vi "RUSHArmControl.vi"(1 "In Cluster":T3) -> (0 "Out Cluster":T2)   [LabVIEW 2012]
uses:
  <vilib>/Rock Robotics/WPI/Relay/WPI_RelayValue.ctl
panel:
  in  "Setpoint P Gain":dbl=2.0
  in  "Manual P Gain":dbl=2.0
  in  "Vision P Gain":dbl=0.75
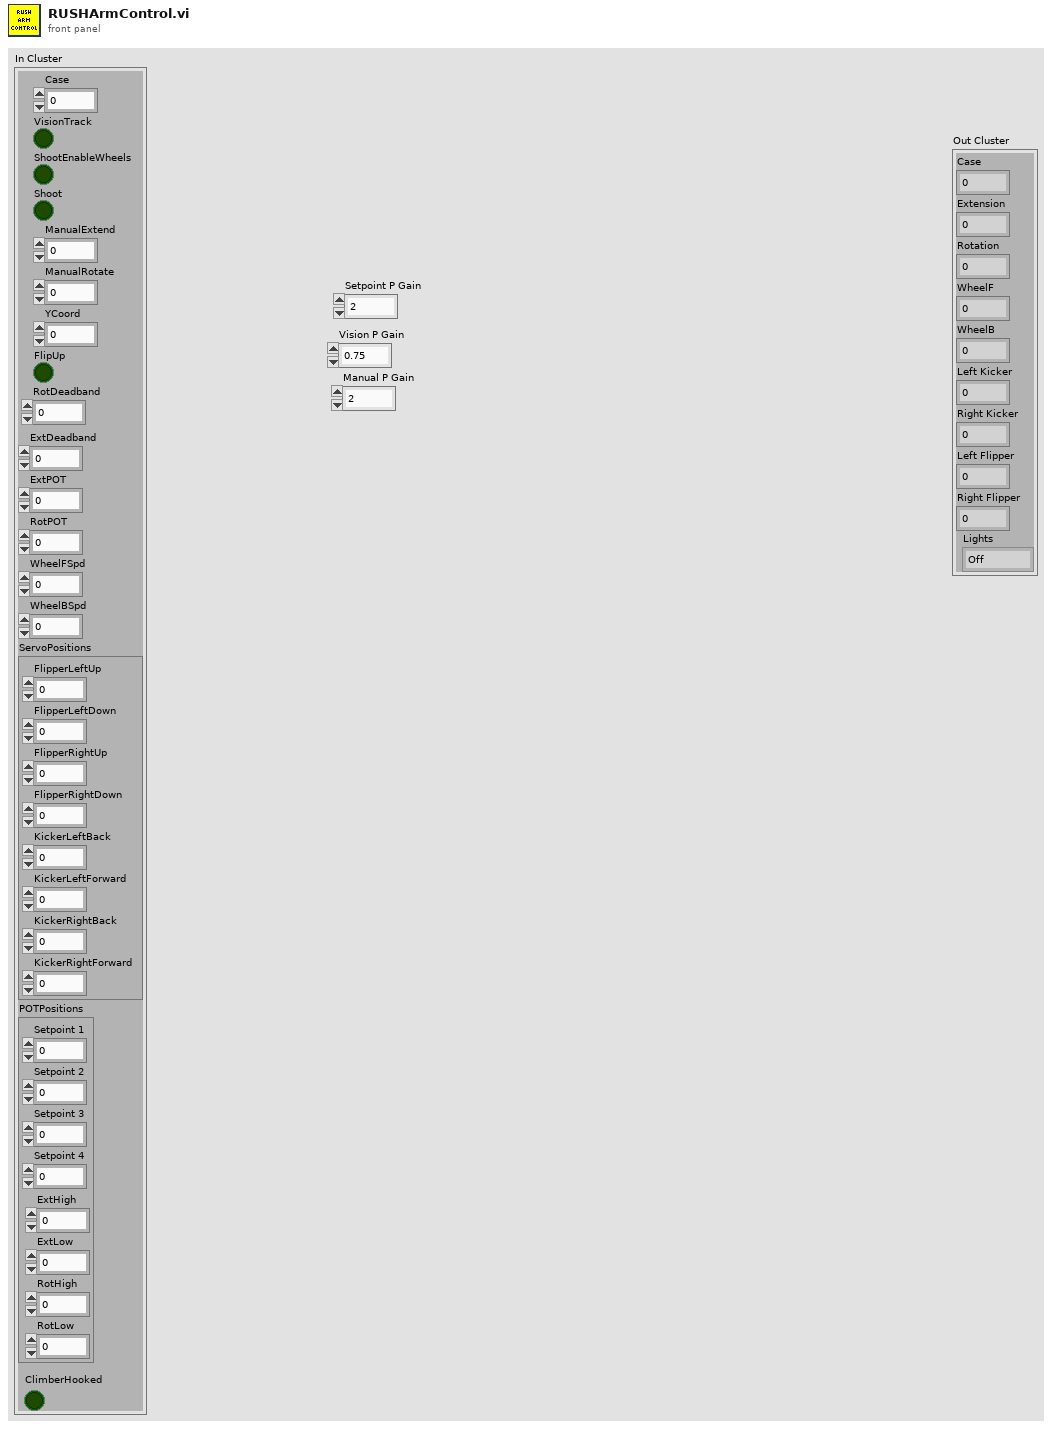
[diagram p1: front panel]
types:
  T1 = typedef "WPI_RelayValue.ctl" = enum16{"Off", "On", "Forward", "Reverse"}
  T2 = cluster{"Case":dbl, "Extension":dbl, "Rotation":dbl, "WheelF":dbl, "WheelB":dbl, "Left Kicker":dbl, "Right Kicker":dbl, "Left Flipper":dbl, "Right Flipper":dbl, "Lights":T1}
  T3 = cluster{"Case":dbl, "VisionTrack":bool, "ShootEnableWheels":bool, "Shoot":bool, "ManualExtend":dbl, "ManualRotate":dbl, "YCoord":dbl, "FlipUp":bool, "RotDeadband":dbl, "ExtDeadband":dbl, "ExtPOT":dbl, "RotPOT":dbl, "WheelFSpd":dbl, "WheelBSpd":dbl, "ServoPositions":cluster{"FlipperLeftUp":dbl, "FlipperLeftDown":dbl, "FlipperRightUp":dbl, "FlipperRightDown":dbl, "KickerLeftBack":dbl, "KickerLeftForward":dbl, "KickerRightBack":dbl, "KickerRightForward":dbl}, "POTPositions":cluster{"Setpoint 1":dbl, "Setpoint 2":dbl, "Setpoint 3":dbl, "Setpoint 4":dbl, "RotLow":dbl, "RotHigh":dbl, "ExtLow":dbl, "ExtHigh":dbl}, "ClimberHooked":bool}
  T4 = cluster{"FlipperLeftUp":dbl, "FlipperLeftDown":dbl, "FlipperRightUp":dbl, "FlipperRightDown":dbl, "KickerLeftBack":dbl, "KickerLeftForward":dbl, "KickerRightBack":dbl, "KickerRightForward":dbl}
  T5 = cluster{"Setpoint 1":dbl, "Setpoint 2":dbl, "Setpoint 3":dbl, "Setpoint 4":dbl, "RotLow":dbl, "RotHigh":dbl, "ExtLow":dbl, "ExtHigh":dbl}
  T6 = cluster{"t":dbl, "y":dbl, "y":dbl, "Output":dbl, "Output":dbl, "KickerLeftBack":dbl, "KickerRightBack":dbl, "FlipperLeftDown":dbl, "FlipperRightDown":dbl, "RelayValue":T1}
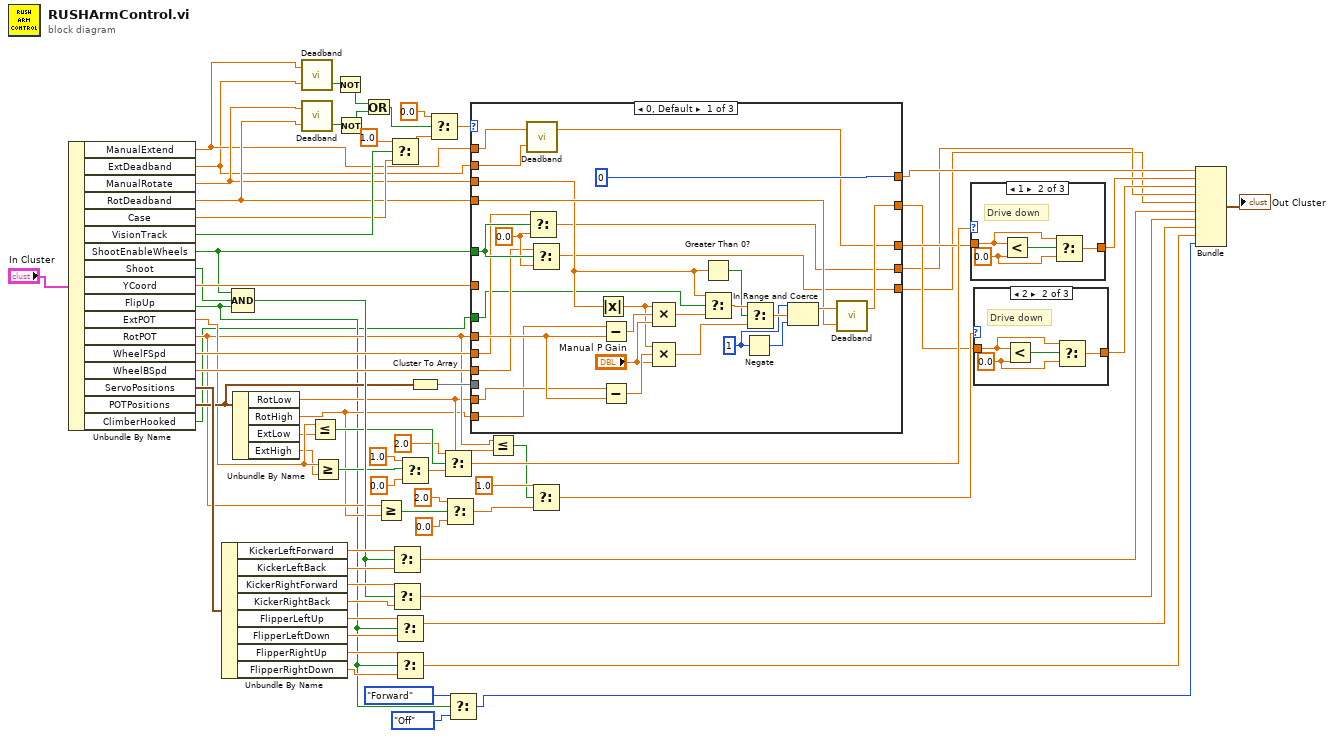
[diagram p0: block diagram]
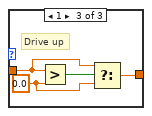
[diagram p3: hidden frame]
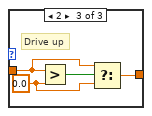
[diagram p5: hidden frame]
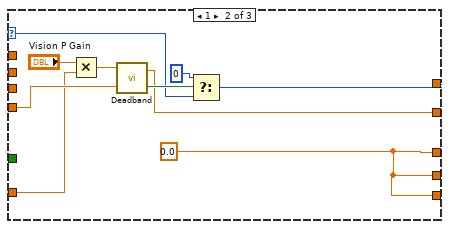
[diagram p6: hidden frame]
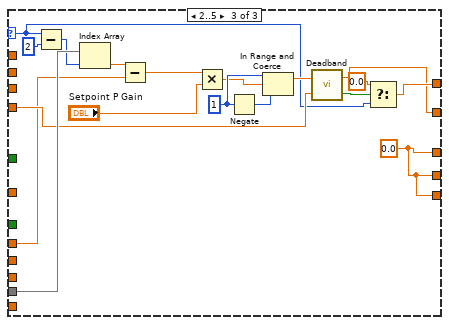
[diagram p7: hidden frame]
diagram:
  n1 = Unbundle By Name("In Cluster") -> ("ManualExtend"=w55:dbl, "ExtDeadband"=w54:dbl, "ManualRotate"=w56:dbl, "RotDeadband"=w58:dbl, "Case"=w59:dbl, "VisionTrack"=w60:bool, "ShootEnableWheels"=w49:bool, "Shoot"=w50:bool, "YCoord"=w57:dbl, "FlipUp"=w5:bool, "ExtPOT"=w32:dbl, "RotPOT"=w20:dbl, "WheelFSpd"=w53:dbl, "WheelBSpd"=w52:dbl, "ServoPositions"=w51:T4, "POTPositions"=w39:T5, "ClimberHooked"=w3:bool)
  n2 = Unbundle By Name(w51) -> ("KickerLeftForward"=w48:dbl, "KickerLeftBack"=w47:dbl, "KickerRightForward"=w46:dbl, "KickerRightBack"=w45:dbl, "FlipperLeftUp"=w43:dbl, "FlipperLeftDown"=w41:dbl, "FlipperRightUp"=w42:dbl, "FlipperRightDown"=w40:dbl)
  n3 = Compound Arithmetic op=AND(w49, w50, w5) -> (w44:bool)
  n4 = Unbundle By Name(w39) -> ("RotLow"=w19:dbl, "RotHigh"=w18:dbl, "ExtLow"=w31:dbl, "ExtHigh"=w30:dbl)
  n5 = call "Deadband.vi"("Deadband"=w54, "Input"=w55) -> ("In Deadband"=w65:bool)  [unwired: 1 out]
  n6 = call "Deadband.vi"("Deadband"=w58, "Input"=w56) -> ("In Deadband"=w64:bool)  [unwired: 1 out]
  n7 = Less Or Equal?(x=w32, y=w31) -> (x <= y?=w33:bool)
  n8 = Greater Or Equal?(x=w32, y=w30) -> (x >= y?=w37:bool)
  n9 = Not(x=w65) -> (.not. x?=w62:bool)
  n10 = Not(x=w64) -> (.not. x?=w63:bool)
  n11 = Or(x=w62, y=w63) -> (x .or. y?=w61:bool)
  n12 = Greater Or Equal?(x=w20, y=w18) -> (x >= y?=w21:bool)
  n13 = Select(t=1.0, s=w60, f=w59) -> (s? t:f=w67:dbl)
  n14 = Select(t=w48, s=w44, f=w47) -> (s? t:f=w10:dbl)
  n15 = Select(t=w46, s=w44, f=w45) -> (s? t:f=w9:dbl)
  n16 = Select(t=w43, s=w5, f=w41) -> (s? t:f=w8:dbl)
  n17 = Select(t=w42, s=w5, f=w40) -> (s? t:f=w7:dbl)
  n18 = Select(t=1.0, s=w37, f=0.0) -> (s? t:f=w34:dbl)
  n19 = Cluster To Array(cluster=w39) -> (array=w38:dbl[])
  n20 = Select(t=0.0, s=w61, f=w67) -> (s? t:f=w70:dbl)
  n21 = Select(t=2.0, s=w33, f=w34) -> (s? t:f=w28:dbl)
  n22 = Select(t=2.0, s=w21, f=0.0) -> (s? t:f=w24:dbl)
  n23 = Select(t=WPI_RelayValue."Forward" ("RelayValue"), s=w5, f=WPI_RelayValue."Off" ("RelayValue")) -> (s? t:f=w1:T1)
  n24 = case shown="0, Default" w70 {
    selector: w70 -> [_ w104 w113]
    tunnel: w58 -> [w84 w107 w117]
    tunnel: w57 -> [_ w106 _]
    tunnel: [0 ("t") w102 w112] -> w15
    tunnel: [w82 w101 w111] -> w16
    tunnel: w20 -> [w87 _ w116]
    tunnel: w19 -> [w86 _ _]
    tunnel: w18 -> [w85 _ _]
    tunnel: w56 -> [w83 _ _]
    tunnel: w55 -> [w80 _ _]
    tunnel: w54 -> [w79 _ _]
    tunnel: [w78 w100 w110] -> w27
    tunnel: w49 -> [w77 _ _]
    tunnel: w53 -> [w75 _ _]
    tunnel: w52 -> [w74 _ _]
    tunnel: [w73 w100 w110] -> w12
    tunnel: [w72 w100 w110] -> w11
    tunnel: w38 -> [_ _ w126]
    tunnel: w3 -> [w71 _ _]
    frame 0, Default {
      w76 = 0.0 ("f")
      w89 = 1
      n25 = call "Deadband.vi"("Deadband"=w79, "Input"=w80) -> ("Output"=w78:dbl)  [unwired: 1 out]
      n26 = Select(t=w75, s=w77, f=w76) -> (s? t:f=w73:dbl)
      n27 = Select(t=w74, s=w77, f=w76) -> (s? t:f=w72:dbl)
      n28 = Absolute Value(x=w83) -> (abs(x)=w93:dbl)
      n29 = Subtract(x=w85, y=w87) -> (x-y=w99:dbl)
      n30 = Subtract(x=w86, y=w87) -> (x-y=w98:dbl)
      n31 = Compound Arithmetic op=MULTIPLY(w93, w99, "Manual P Gain") -> (w96:dbl)
      n32 = Compound Arithmetic op=MULTIPLY(w93, w98, "Manual P Gain") -> (w94:dbl)
      n33 = Greater Than 0?(x=w83) -> (x > 0?=w92:bool)
      n34 = Select(t=w83, s=w71, f=w96) -> (s? t:f=w95:dbl)
      n35 = Negate(x=w89) -> (-x=w90:i32)
      n36 = Select(t=w95, s=w92, f=w94) -> (s? t:f=w91:dbl)
      n37 = In Range and Coerce(upper limit=w89, x=w91, lower limit=w90) -> (coerced(x)=w88:dbl)  [unwired: 1 out]
      n38 = call "Deadband.vi"("Deadband"=w84, "Input"=w88) -> ("Output"=w82:dbl)  [unwired: 1 out]
    }
    frame 1 {
      w100 = 0.0 ("Output")
      n39 = Multiply(x="Vision P Gain", y=w106) -> (x*y=w108:dbl)
      n40 = call "Deadband.vi"("Deadband"=w107, "Input"=w108) -> ("In Deadband"=w105:bool, "Output"=w101:dbl)
      n41 = Select(t=0, s=w105, f=w104) -> (s? t:f=w102:i32)
    }
    frame 2..5 {
      w110 = 0.0 ("Output")
      w120 = 1
      n42 = Subtract(x=w113, y=2) -> (x-y=w125:i32)
      n43 = Index Array(array=w126, index=w125) -> (element=w124:dbl)
      n44 = Subtract(x=w124, y=w116) -> (x-y=w123:dbl)
      n45 = Multiply(x=w123, y="Setpoint P Gain") -> (x*y=w119:dbl)
      n46 = Negate(x=w120) -> (-x=w121:i32)
      n47 = In Range and Coerce(upper limit=w120, x=w119, lower limit=w121) -> (coerced(x)=w118:dbl)  [unwired: 1 out]
      n48 = call "Deadband.vi"("Deadband"=w117, "Input"=w118) -> ("In Deadband"=w115:bool, "Output"=w111:dbl)
      n49 = Select(t=0.0, s=w115, f=w113) -> (s? t:f=w112:dbl)
    }
  }
  n50 = Less Or Equal?(x=w20, y=w19) -> (x <= y?=w25:bool)
  n51 = Select(t=1.0, s=w25, f=w24) -> (s? t:f=w17:dbl)
  n52 = case shown="1" w28 {
    tunnel: w27 -> [w128 w130 w134]
    tunnel: [w128 w129 w133] -> w14
    frame 0, Default {
      # "All good"
    }
    frame 1 {
      w131 = 0.0 ("y")
      # "Drive down"
      n53 = Less?(x=w130, y=w131) -> (x < y?=w132:bool)
      n54 = Select(t=w130, s=w132, f=w131) -> (s? t:f=w129:dbl)
    }
    frame 2 {
      w135 = 0.0 ("y")
      # "Drive up"
      n55 = Greater?(x=w134, y=w135) -> (0:w136:bool)
      n56 = Select(t=w134, s=w136, f=w135) -> (s? t:f=w133:dbl)
    }
  }
  n57 = case shown="2" w17 {
    tunnel: w16 -> [w137 w139 w143]
    tunnel: [w137 w138 w142] -> w13
    frame 0, Default {
      # "All good"
    }
    frame 2 {
      w140 = 0.0 ("y")
      # "Drive down"
      n58 = Less?(x=w139, y=w140) -> (x < y?=w141:bool)
      n59 = Select(t=w139, s=w141, f=w140) -> (s? t:f=w138:dbl)
    }
    frame 1 {
      w144 = 0.0 ("y")
      # "Drive up"
      n60 = Greater?(x=w143, y=w144) -> (0:w145:bool)
      n61 = Select(t=w143, s=w145, f=w144) -> (s? t:f=w142:dbl)
    }
  }
  n62 = Bundle("t"=w15, "y"=w14, "y"=w13, "Output"=w12, "Output"=w11, "KickerLeftBack"=w10, "KickerRightBack"=w9, "FlipperLeftDown"=w8, "FlipperRightDown"=w7, "RelayValue"=w1) -> (→"Out Cluster":T6)  [unwired: 1 in]
